vi "create debug configuration.vi"() -> (0 "error out":errorcluster, 1 "engine dvr":refnum<data-value>, 2 "mapping dvr":refnum<data-value>, 3 "engine configuration out":refnum<class "engine configuration.lvclass">)   [LabVIEW 2013, in "PL Framework Configuration Tool.lvlib" / "Engine Mappings.lvclass"]
uses:
  Engine Mappings.lvclass
  <vilib>/NI/Module Execution Interface/Engine Configuration/engine configuration.lvclass
  Engine Parent/Engine Parent Editor Node.lvclass
  <vilib>/CEF_TreeControl/Node/NISE_CEF_Node.lvclass/NISE_CEF_Node.ctl
  <vilib>/CEF_TreeControl/Node/ReadChildren.vi
  <vilib>/NI/Tag Bus/tag/tag descriptor.lvclass
  <vilib>/CEF_TreeControl/Node/NISE_CEF_Node.lvclass
  <vilib>/NI/Tag Bus/tag/Data Type.ctl
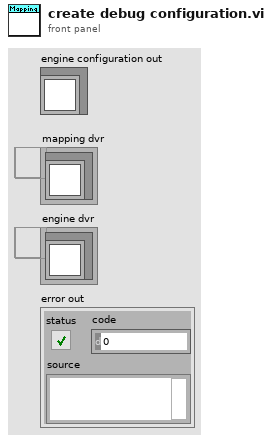
[diagram p1: front panel]
types:
  T1 = typedef "NISE_CEF_Node.lvclass/NodeRef.ctl" = refnum<data-value>
  T2 = typedef "tag bus.lvlib/tag descriptor.lvclass/Data Type.ctl" = enum16{"Double", "Single", "I64", "I32", "I16", "I8", "U64", "U32", "U16", "U8", "Boolean", "String", "Array of Double", "Array of Single", "Array of I64", "Array of I32", "Array of I16", "Array of I8", "Array of U64", "Array of U32", "Array of U16", "Array of U8", "Array of Boolean", "Array of String"}
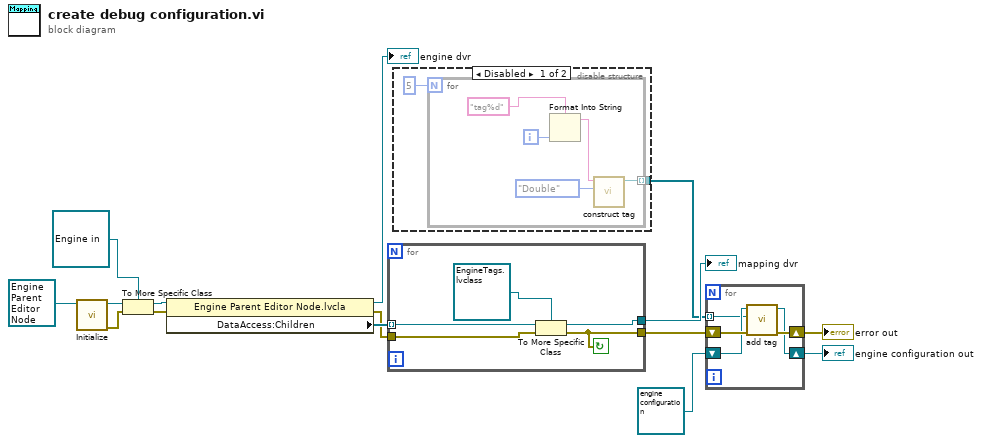
[diagram p0: block diagram]
diagram:
  n1 = call-dynamic "Initialize.vi"("Engine in"=refnum<class "Engine Parent Editor Node.lvclass"> refnum) -> ("error out"=w14:errorcluster, "data value reference"=w11:T1)  [unwired: 8 in, 1 out]
  n2 = To More Specific Class(target class=refnum<data-value> refnum ("data value reference"), reference=w11, error in=w14) -> (specific class reference=w10:refnum<data-value>, error out=w13:errorcluster)
  n3 = property class="Engine Parent Editor Node.lvcla"(reference=w10, error in=w13) -> (reference out=→"engine dvr":refnum<data-value>, error out=w1:errorcluster, "DataAccess:Children"=w7:T1[])
  n4 = for {
    tunnel: [w17] -> w15
    tunnel: [w19] -> w12
    tunnel: w7 -> [w18] mode=indexing
    tunnel: w1 -> [w16]
    stop <- w17 continue-if-true
    n5 = To More Specific Class(target class=refnum<data-value> refnum ("data value reference"), reference=w18, error in=w16) -> (specific class reference=w19:refnum<data-value>, error out=w17:errorcluster)
  }
  "mapping dvr" <- w12
  n6 = disable-structure shown="Disabled" {
    disable-tunnel: [w21 _] -> w4
    frame Disabled {
      n7 = for {
        N: 5 -> [_]
        tunnel: [w23] -> w21 mode=indexing
        i -> [w27]
        n8 = Format Into String(format string="tag%d", w27) -> (resulting string=w25:string)  [unwired: 2 in, 1 out]
        n9 = call <vilib>:"construct tag.vi"("data type"=Data_Type."Double", "name"=w25) -> ("system tag out"=w23:refnum<class "tag descriptor.lvclass">)  [unwired: 9 in]
      }
    }
    frame Enabled {
    }
  }
  n10 = for {
    shift-right: [w30] -> w2
    shift-left: refnum<class "engine configuration.lvclass"> refnum ("engine configuration.lvclass") -> [w29]
    shift-right: [w32] -> w3
    shift-left: w15 -> [w31]
    tunnel: w4 -> [w28] mode=indexing
    n11 = call <vilib>:"add tag.vi"("error in"=w31, "tag descriptor"=w28, "engine configuration in"=w29) -> ("error out"=w32:errorcluster, "engine configuration out"=w30:refnum<class "engine configuration.lvclass">)  [unwired: 7 in]
  }
  "error out" <- w3
  "engine configuration out" <- w2
